vi "hp3458A.vi"() -> ()   [LabVIEW 2015]
panel:
  out "VISA out":refnum<visa-resource-name>
  out "read buffer":string
  out "return count 2":u32
  out "error out":errorcluster
  in  "byte count":u32
  in  "VISA in":refnum<visa-resource-name>
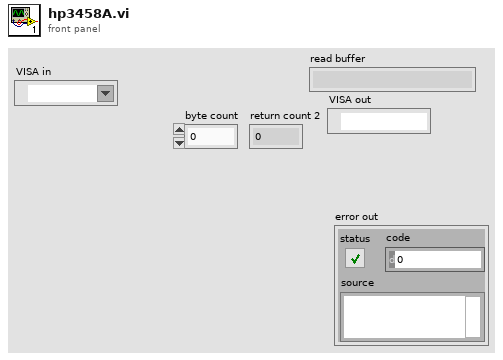
[diagram p1: front panel]
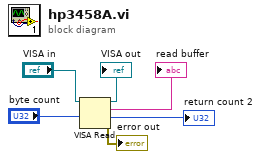
[diagram p0: block diagram]
diagram:
  n1 = VISA Read(VISA resource name="VISA in", byte count="byte count") -> (VISA resource name out=→"VISA out":refnum<visa-resource-name>, read buffer=→"read buffer":string, return count=→"return count 2":u32, error out=→"error out":errorcluster)  [unwired: 1 in]
